vi "Cannon Get.vi"(1 "Eject?":bool, 2 "Throttle":dbl) -> ()   [LabVIEW 2012]
uses:
  Cannon Global Data.vi
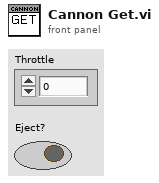
[diagram p1: front panel]
types:
  T1 = cluster{"Throttle":dbl, "RPM":dbl, "Motor VBus":dbl}
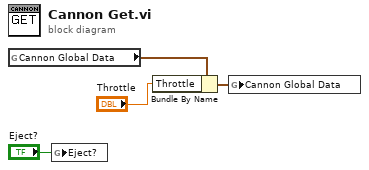
[diagram p0: block diagram]
diagram:
  n1 = global read "Cannon Global Data.vi" "Cannon Global Data"() -> (w3:T1)
  n2 = global write "Cannon Global Data.vi" "Eject?"("Eject?") -> ()
  n3 = Bundle By Name(cluster=w3, "Throttle"="Throttle") -> (w4:T1)
  n4 = global write "Cannon Global Data.vi" "Cannon Global Data"(w4) -> ()
